vi "time-sec-to-time-str-DEC.vi"(1 "Numeric":dbl format="%.1f") -> (0 "formatted-str":string)   [LabVIEW 2019]
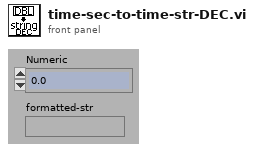
[diagram p1: front panel]
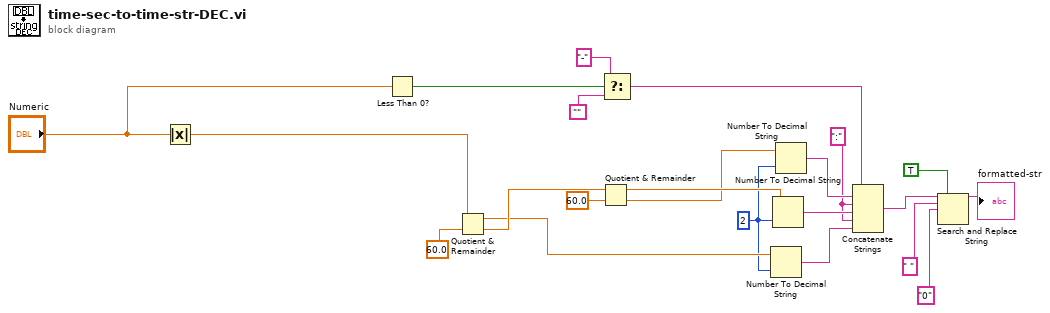
[diagram p0: block diagram]
diagram:
  w5 = i16 2 ("width (-)")
  w15 = ":" ("string")
  n1 = Absolute Value(x="Numeric") -> (abs(x)=w2:dbl)
  n2 = Less Than 0?(x="Numeric") -> (x < 0?=w4:bool)
  n3 = Quotient & Remainder(x=w2, y=60.0) -> (x-y*floor(x/y)=w7:dbl, floor(x/y)=w14:dbl)
  n4 = Quotient & Remainder(x=w14, y=60.0) -> (x-y*floor(x/y)=w12:dbl, floor(x/y)=w11:dbl)
  n5 = Select(t="-" ("string"), s=w4, f="") -> (s? t:f=w10:string)
  n6 = Number To Decimal String(number=w7, width (-)=w5) -> (decimal integer string=w6:string)
  n7 = Number To Decimal String(number=w12, width (-)=w5) -> (decimal integer string=w20:string)
  n8 = Number To Decimal String(number=w11, width (-)=w5) -> (decimal integer string=w21:string)
  n9 = Concatenate Strings(w10, w21, w15, w20, w15, w6) -> (w19:string)
  n10 = Search and Replace String(replace all?=TRUE ("replace all? (F)"), input string=w19, search string=" ", replace string="0" ("replace string (\"\")")) -> (result string=→"formatted-str":string)  [unwired: 4 in, 3 out]
